vi "GLOBAL XYZ STAGE POSITION.vi"() -> ()   [LabVIEW 2018]
panel:
  out "XYZ STAGE POSITION":T1={"X"=4.4501529999999996e-05, "Y"=5.550153e-05, "Z"=5.5500255e-05} {"Z" format="%_6f"; "X" format="%_6f"; "Y" format="%_6f"}
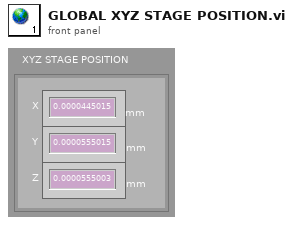
[diagram p1: front panel]
types:
  T1 = cluster{"X":dbl[unit], "Y":dbl[unit], "Z":dbl[unit]}
diagram:
